vi "FIR Narrowband Filter (DBL).vi"(2 "IFIR Coefficients":T1 {"Image Suppressor" format="%0.2e"; "Model Filter" format="%0.2e"}, 3 "X":dbl[](array[numeric])) -> (0 "error":i32, 1 "Filtered X":dbl[](array[numeric]))   [LabVIEW 2017, in "NI_AALBase.lvlib"]
doc: "Filters the input sequence <B>X</B> using the interpolated FIR (IFIR) filter specified by <B>IFIR Coefficients</B>."
uses:
  NI_AALBase.lvlib
  lvanlys.dll
panel:
  # "FIR Narrowband Filter"
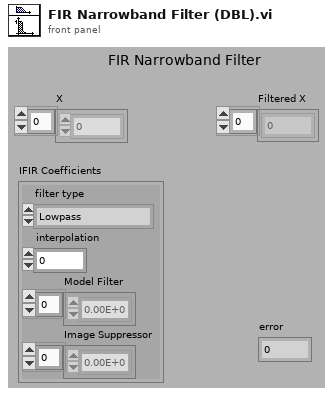
[diagram p1: front panel]
types:
  T1 = cluster{"filter type":enum32{"Lowpass", "Highpass", "Bandpass", "Bandstop", "Wideband-Lowpass", "Wideband-Highpass"}, "interpolation":i32, "Model Filter":dbl[], "Image Suppressor":dbl[]}
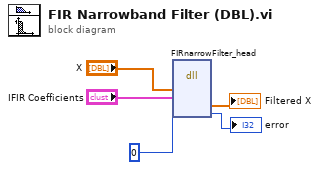
[diagram p0: block diagram]
diagram:
  n1 = dll-call lib="C:/Program Files/National Instruments/LabVIEW 2017/resource/lvanlys.*" fn="FIRnarrowFilter_head"("X"="X", "IFIR Coefficients"="IFIR Coefficients", 0) -> ("Filtered X"=→"Filtered X":dbl[], →"error":i32)  [unwired: 7 in, 2 out]
